vi "IR-Correction_Api.vi"(7 "目標電壓":dbl[](array[numeric])=[2.00487, 2.05982, 2.03994, 2.05787, 1.99765, 2.0512, 2.04107, 2.08625], 8 "Error In":errorcluster, 9 "副邊校正":enum16{"前", "後", "オ", "右", "無"}(ring)=enum."無", 11 "主編校正":enum16{"前", "後", "オ", "右", "無"}(ring)=enum."無") -> (0 "Error Out":errorcluster)   [LabVIEW 2019]
uses:
  <vilib>/Platform/TimedLoop/XDataNode/timing_clust.ctl
  <vilib>/Platform/TimedLoop/XDataNode/nitl_modes.ctl
  <vilib>/Platform/TimedLoop/XDataNode/wakeup.ctl
  <vilib>/addons/control/pid/pid.llb/PID (DBL Array).vi
  <vilib>/platform/TimedLoop/XDataNode/XDataNode.xnode
  <vilib>/addons/control/pid/NI_PID_pid.lvlib
  <vilib>/Platform/TimedLoop/XDataNode/XDNodeRunTimeDep.lvlib
panel:
  in  "Stop":bool
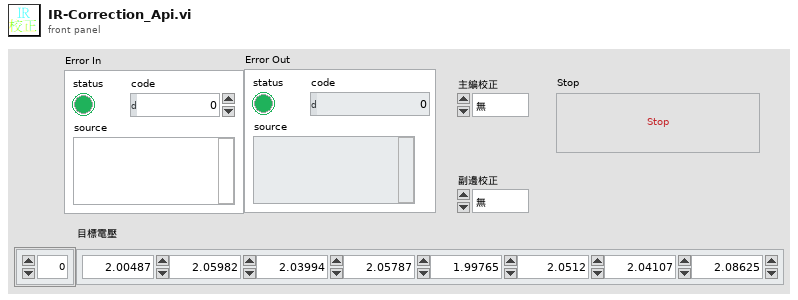
[diagram p1: front panel]
types:
  T1 = cluster{"proportional gain (Kc)":dbl, "integral time (Ti, min)":dbl, "derivative time (Td, min)":dbl}[]
  T2 = typedef "XDNodeRunTimeDep.lvlib/timing_clust.ctl" = cluster{"Expected End [f-1]":u64, "Actual End [f-1]":u64, "Finished Late? [f-1]":bool, "Expected End [i-1]":u64, "Actual End [i-1]":u64, "Finished Late? [i-1]":bool, "Expected Start [i]":u64, "Actual Start [i]":u64, "Expected Start [f]":u64, "Actual Start [f]":u64, "Source Name":string, "Structure Name":string, "Period":i64, "Deadline":i64, "Offset":i64, "Start":i64, "Priority":i32, "Timeout":i32, "Mode":T3, "Wakeup Reason":T4, "Error":errorcluster, "Source Type":string, "Secondary Source Type":string, "Global End Time":u64, "Global Start Time":u64, "Frame Duration":u64, "Iteration Duration":u64, "Assigned CPU":i32, "I/O Scan Engine Mode":u32}
  T3 = typedef "XDNodeRunTimeDep.lvlib/nitl_modes.ctl" = enum32{"No Change", "Process missed periods, maintain original phase", "Discard missed periods, maintain original phase", "Process missed periods, ignore original phase", "Discard missed periods, ignore original phase"}
  T4 = typedef "XDNodeRunTimeDep.lvlib/wakeup.ctl" = enum32{"Normal", "Aborted", "Asynchronous wakeup", "Timing source error", "Timed loop error", "Timeout"}
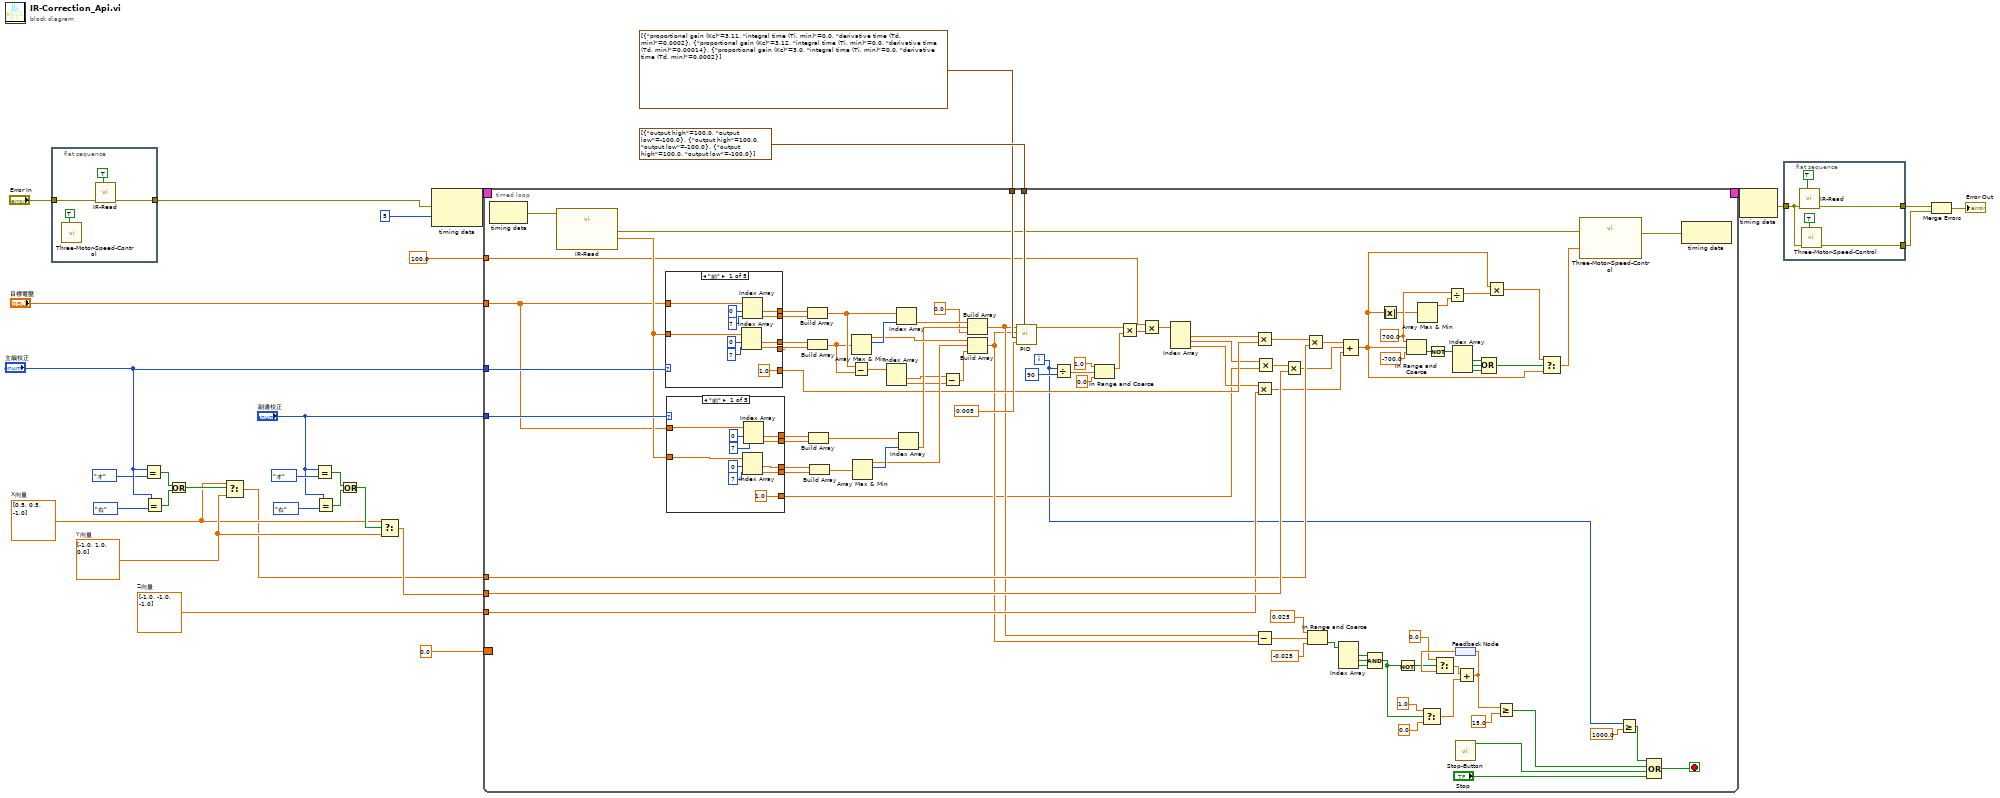
[diagram p0: block diagram]
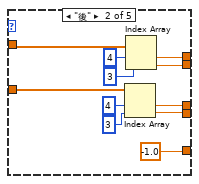
[diagram p2: hidden frame]
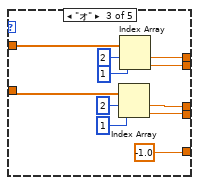
[diagram p3: hidden frame]
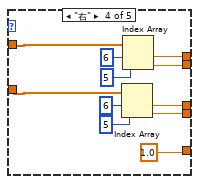
[diagram p4: hidden frame]
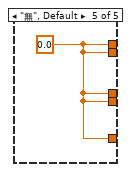
[diagram p5: hidden frame]
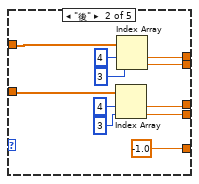
[diagram p6: hidden frame]
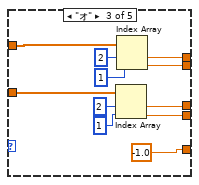
[diagram p7: hidden frame]
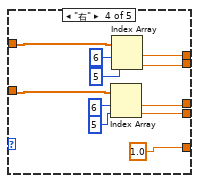
[diagram p8: hidden frame]
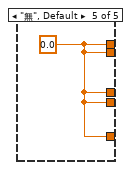
[diagram p9: hidden frame]
diagram:
  w17 = dbl[] [-1.0, -1.0, -1.0]  # Z向量
  w6 = dbl[] [-1.0, 1.0, 0.0]  # Y向量
  w5 = dbl[] [0.5, 0.5, -1.0]  # X向量
  n1 = flat-sequence {
    tunnel: "Error In" -> [w35]
    tunnel: [w34] -> w27
    frame #0 {
      n2 = call "Three-Motor-Speed-Control.vi"("Reset"=TRUE) -> ()  [unwired: 10 in, 1 out]
      n3 = call "IR-Read.vi"("Reset"=TRUE, "Error In"=w35) -> ("Error Out"=w34:errorcluster)  [unwired: 8 in, 1 out]
    }
  }
  n4 = Equal?(x="主編校正", y=enum16{"前", "後", "オ", "右", "無"}."オ") -> (x = y?=w9:bool)
  n5 = Equal?(x="主編校正", y=enum16{"前", "後", "オ", "右", "無"}."右") -> (x = y?=w10:bool)
  n6 = Or(x=w9, y=w10) -> (x .or. y?=w8:bool)
  n7 = Select(t=w5, s=w8, f=w6) -> (s? t:f=w1:dbl[])
  n8 = Equal?(x="副邊校正", y=enum16{"前", "後", "オ", "右", "無"}."オ") -> (x = y?=w21:bool)
  n9 = Equal?(x="副邊校正", y=enum16{"前", "後", "オ", "右", "無"}."右") -> (x = y?=w20:bool)
  n10 = Or(x=w21, y=w20) -> (x .or. y?=w19:bool)
  n11 = Select(t=w5, s=w19, f=w6) -> (s? t:f=w2:dbl[])
  n12 = node-c288(w27, i64 5 ("Period")) -> (w31:T2)
  n13 = timed-loop {
    timing: w31 -> [_]
    timing-out: [_] -> w30
    tunnel: "主編校正" -> [w130]
    tunnel: "目標電壓" -> [w112]
    tunnel: "副邊校正" -> [w114]
    tunnel: cluster{"output high":dbl, "output low":dbl}[] [{"output high"=100.0, "output low"=-100.0}, {"output high"=100.0, "output low"=-100.0}, {"output high"=100.0, "output low"=-100.0}] ("output range") -> [w101]
    tunnel: T1 [{"proportional gain (Kc)"=3.11, "integral time (Ti, min)"=0.0, "derivative time (Td, min)"=0.0002}, {"proportional gain (Kc)"=3.12, "integral time (Ti, min)"=0.0, "derivative time (Td, min)"=0.00014}, {"proportional gain (Kc)"=3.0, "integral time (Ti, min)"=0.0, "derivative time (Td, min)"=0.0002}] ("PID gains") -> [w100]
    tunnel: w17 -> [w90]
    tunnel: w2 -> [w93]
    tunnel: w1 -> [w92]
    border: 0.0 -> [_]
    tunnel: 100.0 ("Numeric") -> [w46]
    i -> [w40]
    stop <- w39 stop-if-true
    w38 = 700.0
    n14 = node-c288() -> (w86:errorcluster)  [unwired: 1 in]
    n15 = call "IR-Read.vi"("Error In"=w86) -> ("Error Out"=w75:errorcluster, "輸出紅外線值"=w113:dbl[])  [unwired: 9 in]
    n16 = case shown="\"前\"" w130 {
      tunnel: w112 -> [w187 w193 w204 w220 _]
      tunnel: w113 -> [w186 w192 w203 w216 _]
      tunnel: [w185 w194 w209 w214 w225] -> w128
      tunnel: [w184 w195 w208 w215 w225] -> w127
      tunnel: [w183 w196 w207 w217 w225] -> w126
      tunnel: [w182 w197 w206 w218 w225] -> w125
      tunnel: [1.0 ("y") -1.0 ("y") -1.0 ("y") 1.0 ("y") w225] -> w97
      frame "前" {
        n17 = Index Array(array=w186, index #1=0 ("index"), index #2=7 ("index")) -> (element #1=w183:dbl, element #2=w182:dbl)
        n18 = Index Array(array=w187, index #1=0 ("index"), index #2=7 ("index")) -> (element #1=w185:dbl, element #2=w184:dbl)
      }
      frame "後" {
        n19 = Index Array(array=w192, index #1=4 ("index"), index #2=3 ("index")) -> (element #1=w196:dbl, element #2=w197:dbl)
        n20 = Index Array(array=w193, index #1=4 ("index"), index #2=3 ("index")) -> (element #1=w194:dbl, element #2=w195:dbl)
      }
      frame "オ" {
        n21 = Index Array(array=w203, index #1=2 ("index"), index #2=1 ("index")) -> (element #1=w207:dbl, element #2=w206:dbl)
        n22 = Index Array(array=w204, index #1=2 ("index"), index #2=1 ("index")) -> (element #1=w209:dbl, element #2=w208:dbl)
      }
      frame "右" {
        n23 = Index Array(array=w216, index #1=6 ("index"), index #2=5 ("index")) -> (element #1=w217:dbl, element #2=w218:dbl)
        n24 = Index Array(array=w220, index #1=6 ("index"), index #2=5 ("index")) -> (element #1=w214:dbl, element #2=w215:dbl)
      }
      frame "無", Default {
        w225 = 0.0 ("Numeric")
      }
    }
    n25 = case shown="\"前\"" w114 {
      tunnel: w112 -> [w137 w143 w157 w171 _]
      tunnel: w113 -> [w136 w142 w158 w169 _]
      tunnel: [w135 w144 w160 w172 w175] -> w115
      tunnel: [w134 w145 w154 w165 w175] -> w116
      tunnel: [w133 w146 w159 w170 w175] -> w117
      tunnel: [w132 w147 w153 w164 w175] -> w118
      tunnel: [1.0 ("y") -1.0 ("y") -1.0 ("y") 1.0 ("y") w175] -> w43
      frame "前" {
        n26 = Index Array(array=w136, index #1=0 ("index"), index #2=7 ("index")) -> (element #1=w133:dbl, element #2=w132:dbl)
        n27 = Index Array(array=w137, index #1=0 ("index"), index #2=7 ("index")) -> (element #1=w135:dbl, element #2=w134:dbl)
      }
      frame "後" {
        n28 = Index Array(array=w142, index #1=4 ("index"), index #2=3 ("index")) -> (element #1=w146:dbl, element #2=w147:dbl)
        n29 = Index Array(array=w143, index #1=4 ("index"), index #2=3 ("index")) -> (element #1=w144:dbl, element #2=w145:dbl)
      }
      frame "オ" {
        n30 = Index Array(array=w158, index #1=2 ("index"), index #2=1 ("index")) -> (element #1=w159:dbl, element #2=w153:dbl)
        n31 = Index Array(array=w157, index #1=2 ("index"), index #2=1 ("index")) -> (element #1=w160:dbl, element #2=w154:dbl)
      }
      frame "右" {
        n32 = Index Array(array=w169, index #1=6 ("index"), index #2=5 ("index")) -> (element #1=w170:dbl, element #2=w164:dbl)
        n33 = Index Array(array=w171, index #1=6 ("index"), index #2=5 ("index")) -> (element #1=w172:dbl, element #2=w165:dbl)
      }
      frame "無", Default {
        w175 = 0.0 ("Numeric")
      }
    }
    n34 = Build Array(w128, w127) -> (w107:dbl[])
    n35 = Build Array(w126, w125) -> (w106:dbl[])
    n36 = Build Array(w115, w116) -> (w120:dbl[])
    n37 = Build Array(w117, w118) -> (w119:dbl[])
    n38 = Array Max & Min(array=w106) -> (max value=w122:dbl, max index (indices)=w124:i32)  [unwired: 2 out]
    n39 = Subtract(x=w107, y=w106) -> (x-y=w105:dbl[])
    n40 = Array Max & Min(array=w119) -> (max value=w109:dbl, max index (indices)=w121:i32)  [unwired: 2 out]
    n41 = Index Array(array=w105) -> (element #1=w104:dbl, element #2=w103:dbl)  [unwired: 2 in]
    n42 = Index Array(array=w107, index=w124) -> (element=w123:dbl)
    n43 = Index Array(array=w120, index=w121) -> (element=w110:dbl)
    n44 = Subtract(x=w104, y=w103) -> (x-y=w102:dbl)
    n45 = Build Array(w123, w110, 0.0 ("element")) -> (w73:dbl[])
    n46 = Build Array(w122, w109, w102) -> (w72:dbl[])
    n47 = call-poly <vilib>:"PID.vi"("output range"=w101, "dt (s)"=0.005, "PID gains"=w100, "process variable"=w72, "setpoint"=w73) -> ("output"=w49:dbl[])  [unwired: 5 in, 1 out]
    n48 = Divide(x=w40, y=90) -> (x/y=w53:dbl)
    n49 = In Range and Coerce(upper limit=1.0, x=w53, lower limit=0.0) -> (coerced(x)=w50:dbl)  [unwired: 1 out]
    n50 = Multiply(x=w49, y=w50) -> (x*y=w47:dbl[])
    n51 = Multiply(x=w46, y=w47) -> (x*y=w48:dbl[])
    n52 = Index Array(array=w48) -> (element #1=w98:dbl, element #2=w96:dbl, element #3=w91:dbl)  [unwired: 3 in]
    n53 = Multiply(x=w98, y=w97) -> (x*y=w95:dbl)
    n54 = Multiply(x=w91, y=w90) -> (x*y=w87:dbl[])
    n55 = Subtract(x=w73, y=w72) -> (x-y=w74:dbl[])
    n56 = Multiply(x=w96, y=w43) -> (x*y=w94:dbl)
    n57 = Multiply(x=w94, y=w93) -> (x*y=w88:dbl[])
    n58 = Multiply(x=w95, y=w92) -> (x*y=w89:dbl[])
    n59 = In Range and Coerce(upper limit=0.025, x=w74, lower limit=-0.025) -> (In Range?=w69:bool[])  [unwired: 1 out]
    n60 = Index Array(array=w69) -> (element #1=w68:bool, element #2=w67:bool, element #3=w66:bool)  [unwired: 3 in]
    n61 = Compound Arithmetic op=ADD(w89, w88, w87) -> (w36:dbl[])
    n62 = Compound Arithmetic op=AND(w68, w67, w66) -> (w60:bool)
    n63 = Absolute Value(x=w36) -> (abs(x)=w37:dbl[])
    n64 = Not(x=w60) -> (.not. x?=w61:bool)
    n65 = In Range and Coerce(upper limit=w38, x=w36, lower limit=-700.0) -> (In Range?=w84:bool[])  [unwired: 1 out]
    n66 = Array Max & Min(array=w37) -> (max value=w44:dbl)  [unwired: 3 out]
    n67 = Select(t=1.0, s=w60, f=0.0) -> (s? t:f=w63:dbl)
    n68 = Not(x=w84) -> (.not. x?=w83:bool[])
    n69 = Divide(x=w38, y=w44) -> (x/y=w77:dbl)
    n70 = Index Array(array=w83) -> (element #1=w82:bool, element #2=w81:bool, element #3=w80:bool)  [unwired: 3 in]
    n71 = feedback #1() -> (w62:dbl)
    n72 = Select(t=0.0, s=w61, f=w62) -> (s? t:f=w58:dbl)
    n73 = call "Stop-Button.vi"() -> ("顯示按下?"=w111:bool)  [unwired: 10 in, 1 out]
    n74 = Add(x=w58, y=w63) -> (x+y=w57:dbl)
    n75 = feedback-in #1(w57) -> ()
    n76 = Compound Arithmetic op=OR(w82, w81, w80) -> (w79:bool)
    n77 = Multiply(x=w36, y=w77) -> (x*y=w76:dbl[])
    n78 = Greater Or Equal?(x=w57, y=15.0) -> (x >= y?=w55:bool)
    n79 = Select(t=w76, s=w79, f=w36) -> (s? t:f=w78:dbl[])
    n80 = call "Three-Motor-Speed-Control.vi"("Error In"=w75, "速度(秒/度)"=w78) -> ("Error Out"=w45:errorcluster)  [unwired: 9 in]
    n81 = Greater Or Equal?(x=w40, y=1000.0) -> (x >= y?=w42:bool)
    n82 = Compound Arithmetic op=OR(w42, w55, w111, "Stop") -> (w39:bool)
    n83 = node-c288(w45) -> ()  [unwired: 1 out]
  }
  n84 = node-c288(w30) -> (w16:errorcluster)
  n85 = flat-sequence {
    tunnel: w16 -> [w230]
    tunnel: [w229] -> w15
    tunnel: [w228] -> w11
    frame #0 {
      n86 = call "IR-Read.vi"("Reset"=TRUE, "Error In"=w230) -> ("Error Out"=w229:errorcluster)  [unwired: 8 in, 1 out]
      n87 = call "Three-Motor-Speed-Control.vi"("Reset"=TRUE, "Error In"=w230) -> ("Error Out"=w228:errorcluster)  [unwired: 9 in]
    }
  }
  n88 = Merge Errors(w15, w11) -> (→"Error Out":errorcluster)
